vi "CRYView In CurLibrary.vi"(8 "sOption":string, 9 "nData":i32, 10 "sData":string, 11 "sAction":string) -> (0 "bResult":bool=TRUE, 1 "pRefList_Out":variant[](array[variant]), 2 "pVIRef_Out":refnum<vi>, 3 "SData_Out":string)   [LabVIEW 2013]
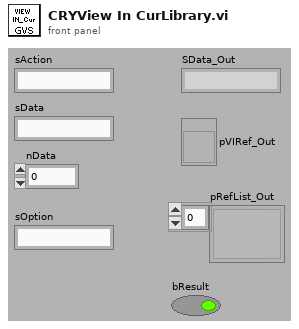
[diagram p1: front panel]
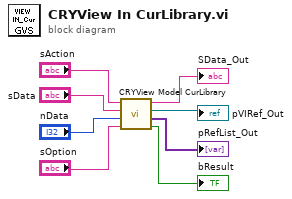
[diagram p0: block diagram]
diagram:
  n1 = call "CRYView Model CurLibrary.vi"("sOption"="sOption", "nData"="nData", "sData"="sData", "sAction"="sAction") -> ("bResult"=→"bResult":bool, "pRefList_Out"=→"pRefList_Out":variant[], "pVIRef_Out"=→"pVIRef_Out":refnum<vi>, "SData_Out"=→"SData_Out":string)  [unwired: 4 in]
